vi "Relay.vi"(8 "error in":errorcluster, 9 "RelayMode":T1, 10 "Line(s)":string="PXIe-6514/port4/line0:2", 11 "DIO":refnum<class "DIO.lvclass">) -> (0 "error out":errorcluster={"status"=TRUE, "code"=1446, "source"="Preserve Run-Time Class in MAL.lvlib:Relay.vi"}, 3 "DIO out":refnum<class "DIO.lvclass">)   [LabVIEW 2019, in "Code Modules.lvlib"]
uses:
  Code Modules.lvlib
  PPLs/Hardware Abstraction.lvlibp/Harware Abstraction/DIO/DIO.lvclass
  RelayMode -Enum.ctl
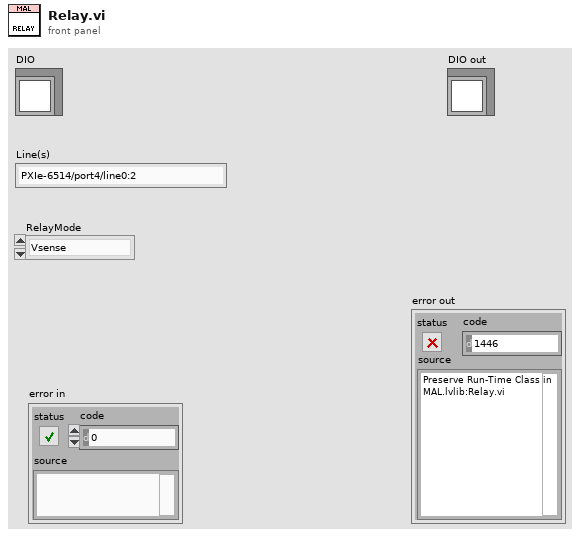
[diagram p1: front panel]
types:
  T1 = typedef "Code Modules.lvlib/RelayMode -Enum.ctl" = enum16{"Vsense", "Thermistor", "ACIR", "HiPOT1", "HiPOT2"}
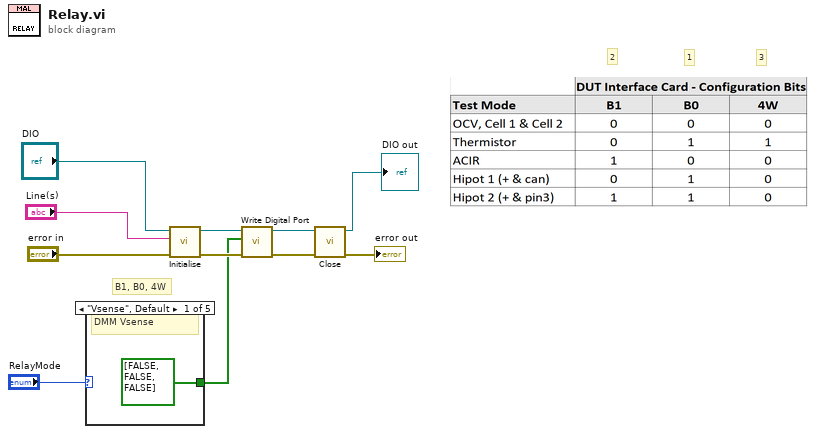
[diagram p0: block diagram]
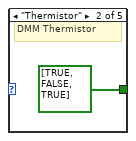
[diagram p2: hidden frame]
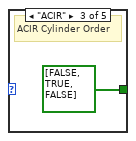
[diagram p3: hidden frame]
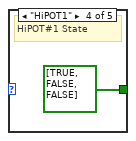
[diagram p4: hidden frame]
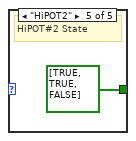
[diagram p5: hidden frame]
diagram:
  # "3"
  # "2"
  # "1"
  # "B1, B0, 4W"
  n1 = case shown="\"Vsense\", Default" "RelayMode" {
    tunnel: [bool[] [FALSE, FALSE, FALSE] bool[] [TRUE, FALSE, TRUE] bool[] [FALSE, TRUE, FALSE] bool[] [TRUE, FALSE, FALSE] bool[] [TRUE, TRUE, FALSE]] -> w1
    frame "Vsense", Default {
      # "DMM Vsense"
    }
    frame "Thermistor" {
      # "DMM Thermistor"
    }
    frame "ACIR" {
      # "ACIR Cylinder Order"
    }
    frame "HiPOT1" {
      # "HiPOT#1 State"
    }
    frame "HiPOT2" {
      # "HiPOT#2 State"
    }
  }
  n2 = call-dynamic "Initialise.vi"("error in (no error)"="error in", "Instrument Ref"="Line(s)", "Instrument in"="DIO") -> ("error out"=w11:errorcluster, "Instrument out"=w5:refnum<class "DIO.lvclass">)  [unwired: 7 in]
  n3 = call-dynamic "Write Digital Port.vi"("error in (no error)"=w11, "Relay Mode"=w1, "DIO in"=w5) -> ("error out"=w10:errorcluster, "DIO out"=w9:refnum<class "DIO.lvclass">)  [unwired: 7 in]
  n4 = call-dynamic "Close.vi"("error in (no error)"=w10, "Instrument in"=w9) -> ("error out"=→"error out":errorcluster, "Instrument out"=→"DIO out":refnum<class "DIO.lvclass">)  [unwired: 8 in]
